vi "02deco_medicion.vi"(1 "medicion":dbl, 2 "caract":u8) -> (0 "Numeric":dbl format="%.2f")   [LabVIEW 2010]
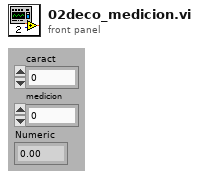
[diagram p1: front panel]
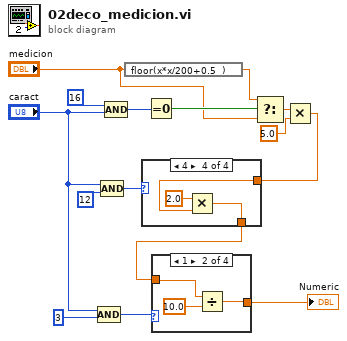
[diagram p0: block diagram]
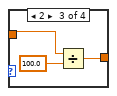
[diagram p3: hidden frame]
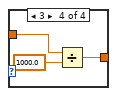
[diagram p4: hidden frame]
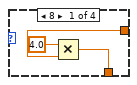
[diagram p5: hidden frame]
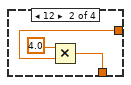
[diagram p6: hidden frame]
diagram:
  n1 = Compound Arithmetic op=AND("caract", u8 3 ("Input")) -> (w3:u8)
  n2 = Compound Arithmetic op=AND("caract", u8 12 ("Input")) -> (w7:u8)
  n3 = Compound Arithmetic op=AND(u8 16, "caract") -> (w8:u8)
  n4 = expression code="floor(x*x/200+0.5  )"("medicion") -> (w2:dbl)
  n5 = Equal To 0?(x=w8) -> (x = 0?=w13:bool)
  n6 = Select(t=w2, s=w13, f="medicion") -> (s? t:f=w11:dbl)
  n7 = Multiply(x=w11, y=5.0) -> (x*y=w9:dbl)
  n8 = case shown="4" w7 {
    tunnel: w9 -> [w18 w21 w22 w25]
    tunnel: [w16 w19 w22 w23] -> w6
    frame 8 {
      n9 = Multiply(x=4.0, y=w18) -> (x*y=w16:dbl)
    }
    frame 12 {
      n10 = Multiply(x=4.0, y=w21) -> (x*y=w19:dbl)
    }
    frame 0, Default {
    }
    frame 4 {
      n11 = Multiply(x=2.0, y=w25) -> (x*y=w23:dbl)
    }
  }
  n12 = case shown="1" w3 {
    tunnel: w6 -> [w26 w29 w32 w35]
    tunnel: [w26 w27 w30 w33] -> w15
    frame 0, Default {
    }
    frame 1 {
      n13 = Divide(x=w29, y=10.0) -> (x/y=w27:dbl)
    }
    frame 2 {
      n14 = Divide(x=w32, y=100.0) -> (x/y=w30:dbl)
    }
    frame 3 {
      n15 = Divide(x=w35, y=1000.0) -> (x/y=w33:dbl)
    }
  }
  "Numeric" <- w15
